vi "getValue.vi"(8 "error in (no error)":errorcluster, 11 "IInteger in":refnum<class "IInteger.lvclass">) -> (0 "error out":errorcluster, 2 "Value out":i32, 3 "IInteger out":refnum<class "IInteger.lvclass">)   [LabVIEW 2022 SP3, in "openDAQ.lvlib" / "daqCoreTypes.lvlib" / "IInteger.lvclass"]
uses:
  <instrlib>/openDAQ/Public/Classes/daqCoreTypes/IInteger/IInteger.lvclass
  C:/Program Files (x86)/National Instruments/LabVIEW 2022/instr.lib/openDAQ/Public/Classes/IBaseObject/IBaseObject.lvclass
  <instrlib>/openDAQ/Public/Classes/IBaseObject/IBaseObject.lvclass/IBaseObject.ctl
  <instrlib>/openDAQ/Public/Classes/IBaseObject/Accessor/Read reference.vi
  <instrlib>/openDAQ/Public/Classes/IBaseObject/Accessor/Write reference.vi
  <instrlib>/openDAQ/Binaries/Windows/x86/copendaq32.dll
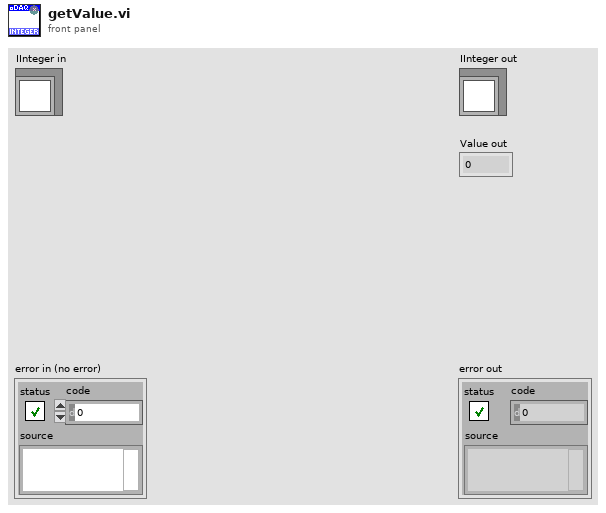
[diagram p1: front panel]
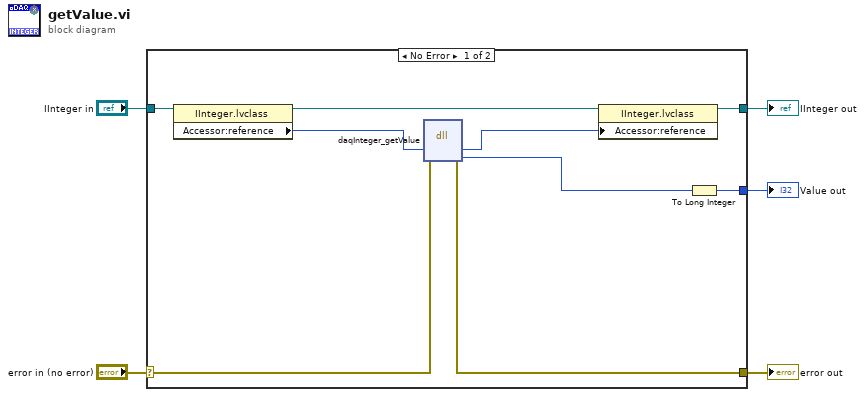
[diagram p0: block diagram]
diagram:
  n1 = case shown="No Error" "error in (no error)" {
    selector: "error in (no error)" -> [w13 w16]
    tunnel: [w12 w16] -> w4
    tunnel: [w10 w15] -> w2
    tunnel: "IInteger in" -> [w14 w15]
    tunnel: [w6 _] -> w1
    frame No Error {
      n2 = property class="IInteger.lvclass"(reference=w14) -> (reference out=w11:refnum<class "IInteger.lvclass">, "Accessor:reference"=w9:i64)  [unwired: 1 in, 1 out]
      n3 = dll-call lib="C:/Program Files (x86)/National Instruments/LabVIEW 2022/instr.lib/openDAQ/Binaries/Windows/x86/copendaq*.*" fn="daqInteger_getValue"(error in=w13, "obj"=w9) -> (error out=w12:errorcluster, "obj"=w8:i64, "value"=w7:i64)  [unwired: 4 in, 1 out]
      n4 = property class="IInteger.lvclass"(reference=w11, "Accessor:reference"=w8) -> (reference out=w10:refnum<class "IInteger.lvclass">)  [unwired: 1 in, 1 out]
      n5 = To Long Integer(number=w7) -> (32bit integer=w6:i32)
    }
    frame Error {
    }
  }
  "error out" <- w4
  "IInteger out" <- w2
  "Value out" <- w1
